vi "Parser_0x51_(SubVI).vi"(8 "error in":errorcluster, 10 "NumberTableParam":i32 format="%0d", 11 "String in":string="!01515B5461626C655D0A466F726D61743D310A4163636573733D726F0A506172616D4E756D3D300A4E616D653D54657374436170747572650A446573633D5465737420636170747572650A547970653D667261637431360A436F6C733D320A526F77733D310A4E656564506172616D507265706172653D790A466F726D61745374723D2534660A85\r") -> (0 "error out":errorcluster, 1 "CheckSummGood":bool, 3 "output cluster":T1)   [LabVIEW 2017, in "LV_Unicorn.lvlib"]
uses:
  LV_Unicorn.lvlib
  Control/unicorn_Table.ctl
panel:
  out "Array":string[][](array[string])
  out "StringOut":string
  out "CalcCheckSumm_U32":u32 format="%02x"
  out "ReciveCheckSumm_U32":i32 format="%x"
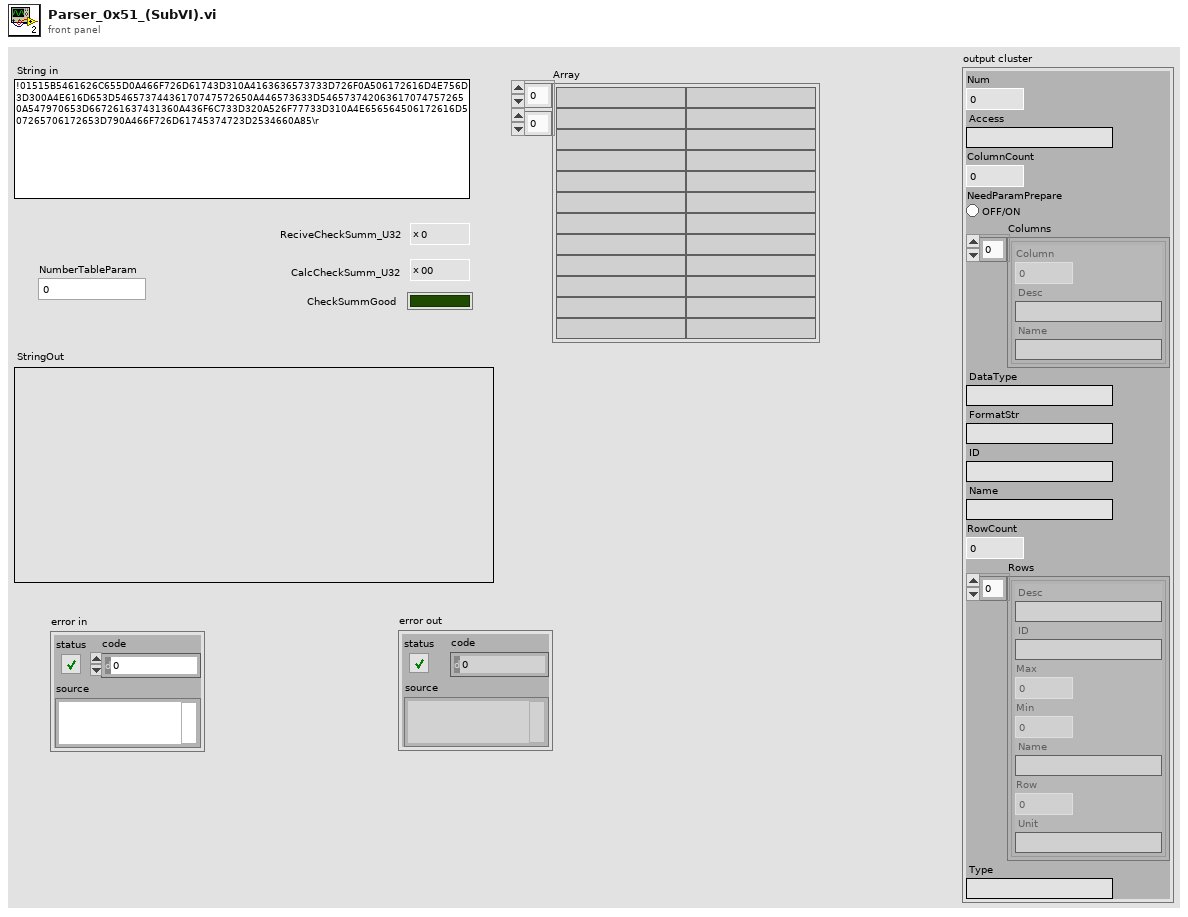
[diagram p1: front panel]
types:
  T1 = cluster{"Num":i32, "Access":string, "ColumnCount":i32, "NeedParamPrepare":bool, "Columns":cluster{"Column":i32, "Desc":string, "Name":string}[], "DataType":string, "FormatStr":string, "ID":string, "Name":string, "RowCount":i32, "Rows":cluster{"Desc":string, "ID":string, "Max":i32, "Min":i32, "Name":string, "Row":i32, "Unit":string}[], "Type":string}
  T2 = cluster{"Desc":string, "ID":string, "Max":i32, "Min":i32, "Name":string, "Row":i32, "Unit":string}[]
  T3 = cluster{"Column":i32, "Desc":string, "Name":string}[]
  T4 = typedef "LV_Unicorn.lvlib/unicorn_Table.ctl" = cluster{"Num":i32, "Access":string, "ColumnCount":i32, "NeedParamPrepare":bool, "Columns":cluster{"Column":i32, "Desc":string, "Name":string}[], "DataType":string, "FormatStr":string, "ID":string, "Name":string, "RowCount":i32, "Rows":cluster{"Desc":string, "ID":string, "Max":i32, "Min":i32, "Name":string, "Row":i32, "Unit":string}[], "Type":string}[]
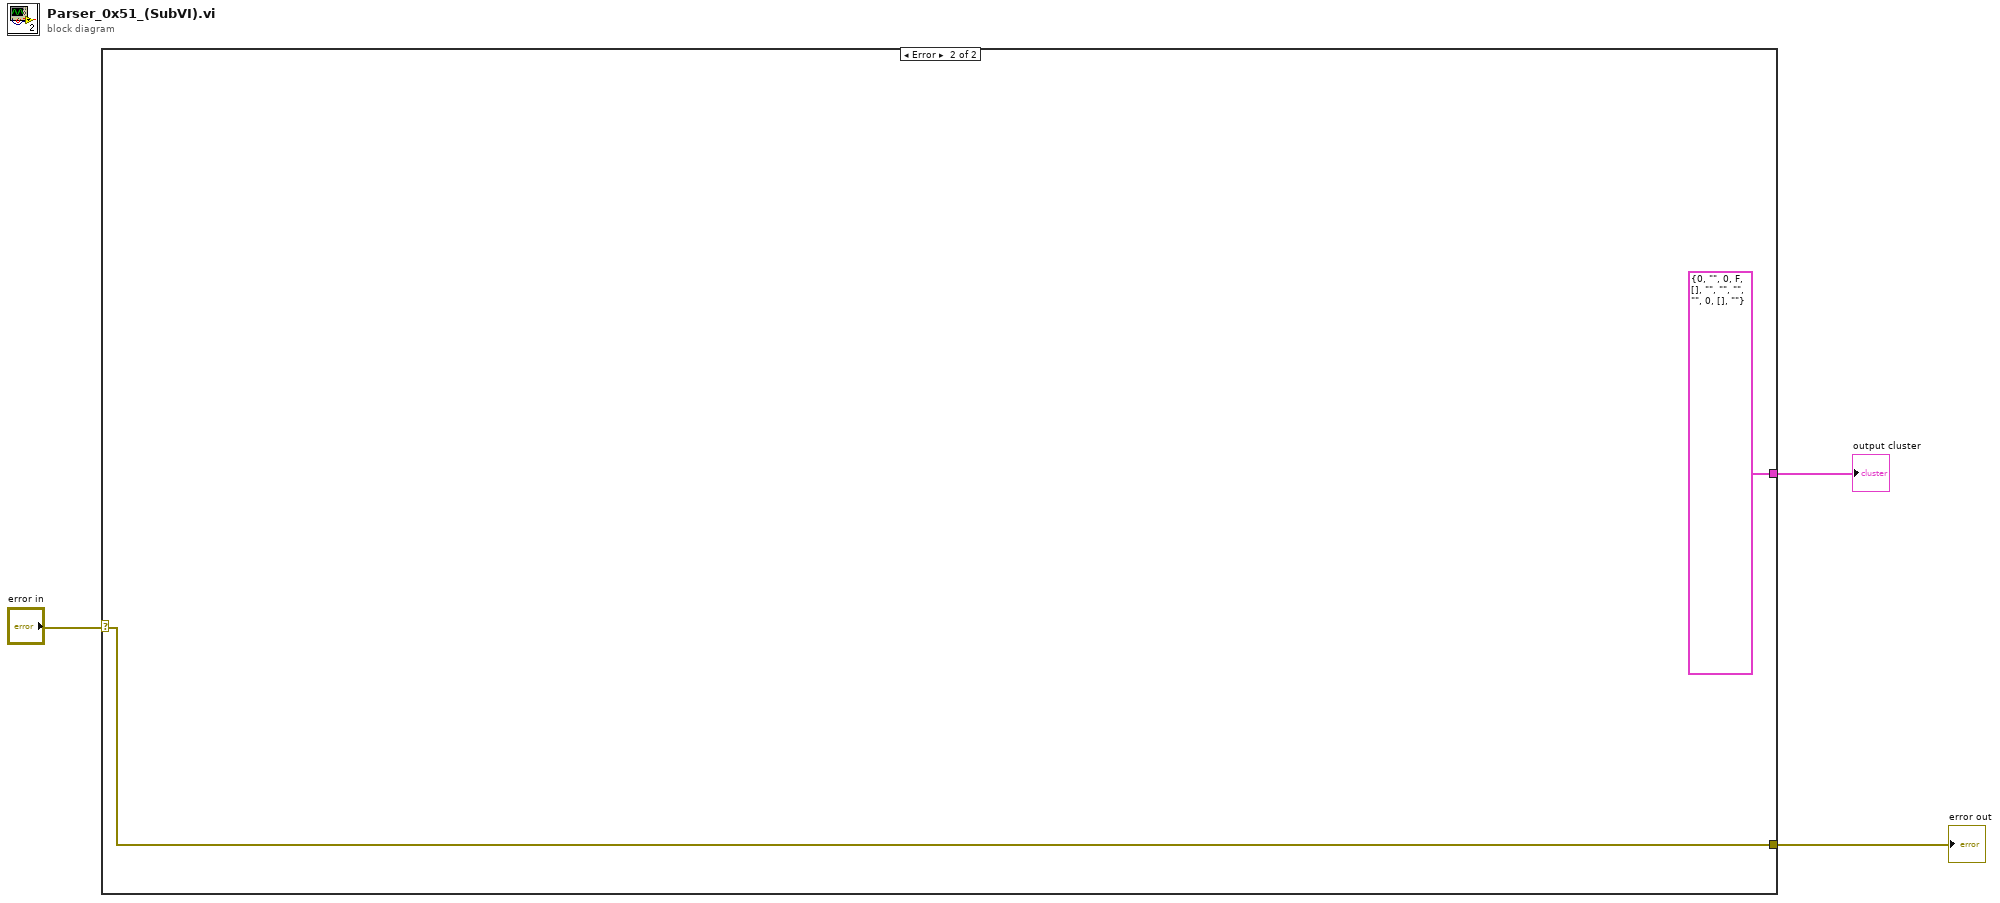
[diagram p0: block diagram]
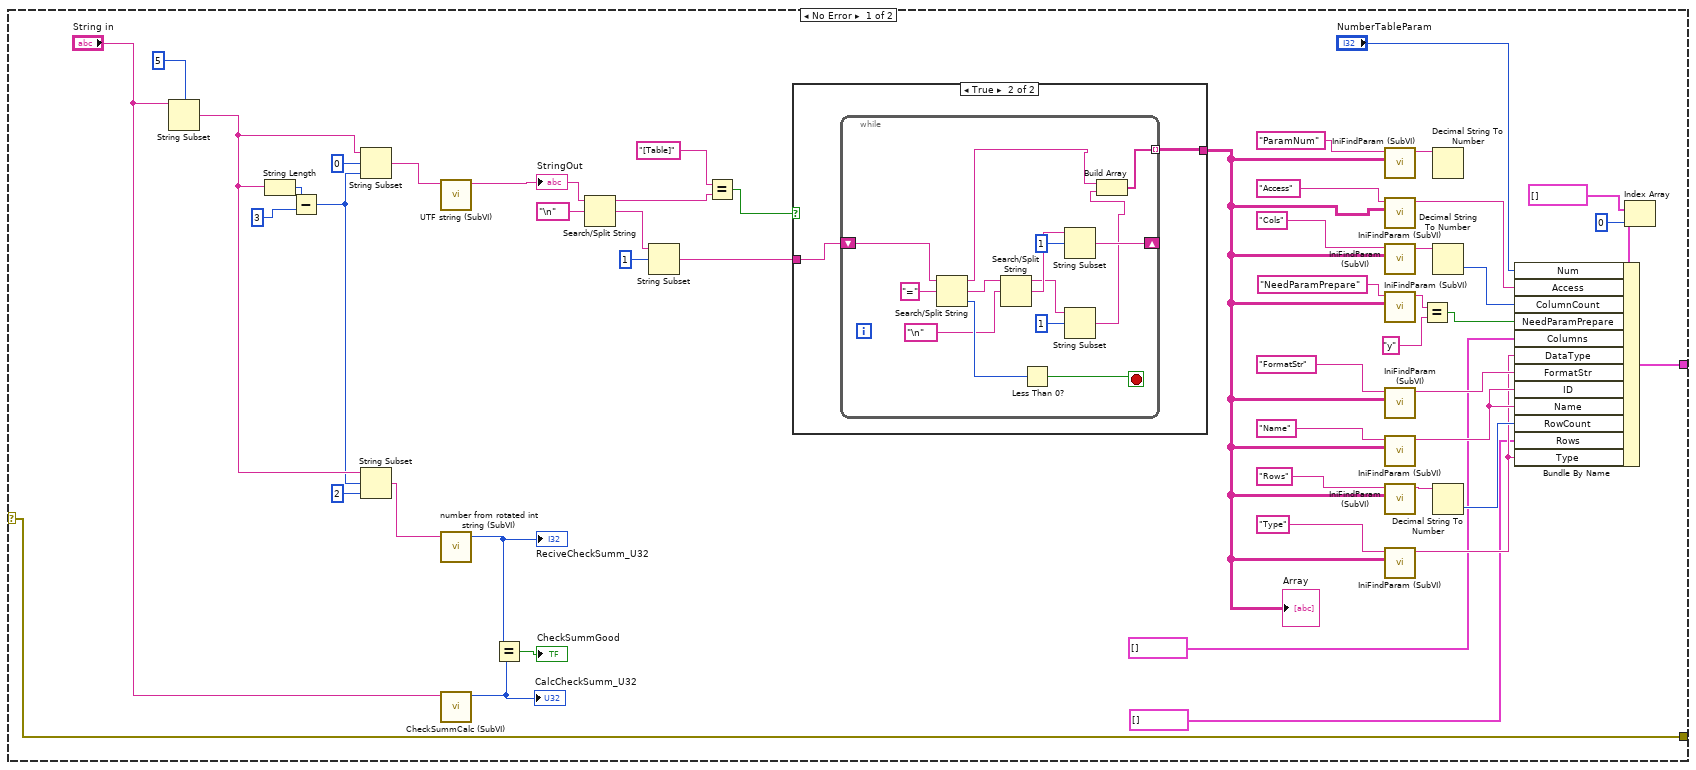
[diagram p2: hidden frame]
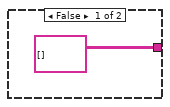
[diagram p3: hidden frame]
diagram:
  n1 = case shown="Error" "error in" {
    selector: "error in" -> [w4 w71]
    tunnel: [w18 T1 {"Num"=0, "Access"="", "ColumnCount"=0, "NeedParamPrepare"=FALSE, "Columns"=[], "DataType"="", "FormatStr"="", "ID"="", "Name"="", "RowCount"=0, "Rows"=[], "Type"=""} ("Cluster - Thin Border")] -> w3
    tunnel: [w4 w71] -> w1
    frame No Error {
      n2 = String Subset(string="String in", offset (0)=5) -> (substring=w44:string)  [unwired: 1 in]
      n3 = String Length(string=w44) -> (length=w47:i32)
      n4 = Subtract(x=w47, y=3) -> (x-y=w43:i32)
      n5 = String Subset(string=w44, offset (0)=0, length (rest)=w43) -> (substring=w45:string)
      n6 = String Subset(string=w44, offset (0)=w43, length (rest)=2 ("length (rest)")) -> (substring=w42:string)
      n7 = call "UTF string (SubVI).vi"("StringIn"=w45) -> ("StringOut"=w40:string)  [unwired: 9 in, 1 out]
      "StringOut" <- w40
      n8 = call "number from rotated int string (SubVI).vi"("String"=w42) -> ("rotated int number"=w51:i32)  [unwired: 2 in, 2 out]
      "ReciveCheckSumm_U32" <- w51
      n9 = call "CheckSummCalc (SubVI).vi"("String in"="String in") -> ("CheckSumm_U32"=w50:u32)  [unwired: 10 in]
      "CalcCheckSumm_U32" <- w50
      n10 = Equal?(x=w51, y=w50) -> (x = y?=→"CheckSummGood":bool)
      n11 = Search/Split String(string=w40, search string/char (-)="\n") -> (substring before match=w35:string, match + rest of string=w38:string)  [unwired: 1 in, 1 out]
      n12 = String Subset(string=w38, offset (0)=1) -> (substring=w33:string)  [unwired: 1 in]
      n13 = Equal?(x="[Table]" ("substring before match"), y=w35) -> (x = y?=w34:bool)
      n14 = case shown="True" w34 {
        tunnel: w33 -> [_ w56]
        tunnel: [string[][] [] w55] -> w9
        frame False {
        }
        frame True {
          n15 = while {
            shift-right: [w65] -> _
            shift-left: w56 -> [w70]
            tunnel: [w57] -> w55 mode=indexing
            stop <- w67 stop-if-true
            n16 = Search/Split String(string=w70, search string/char (-)="=") -> (substring before match=w59:string, match + rest of string=w64:string, offset of match=w68:i32)  [unwired: 1 in]
            n17 = Search/Split String(string=w64, search string/char (-)="\n") -> (substring before match=w60:string, match + rest of string=w62:string)  [unwired: 1 in, 1 out]
            n18 = Less Than 0?(x=w68) -> (x < 0?=w67:bool)
            n19 = String Subset(string=w62, offset (0)=1) -> (substring=w65:string)  [unwired: 1 in]
            n20 = String Subset(string=w60, offset (0)=1) -> (substring=w58:string)  [unwired: 1 in]
            n21 = Build Array(w59, w58) -> (w57:string[])
          }
        }
      }
      "Array" <- w9
      n22 = call "IniFindParam (SubVI).vi"("Array"=w9, "element"="ParamNum") -> ("StringOut"=w16:string)  [unwired: 9 in]
      n23 = call "IniFindParam (SubVI).vi"("Array"=w9, "element"="Access") -> ("StringOut"=w8:string)  [unwired: 9 in]
      n24 = call "IniFindParam (SubVI).vi"("Array"=w9, "element"="Cols") -> ("StringOut"=w28:string)  [unwired: 9 in]
      n25 = call "IniFindParam (SubVI).vi"("Array"=w9, "element"="NeedParamPrepare") -> ("StringOut"=w13:string)  [unwired: 9 in]
      n26 = call "IniFindParam (SubVI).vi"("Array"=w9, "element"="FormatStr") -> ("StringOut"=w20:string)  [unwired: 9 in]
      n27 = call "IniFindParam (SubVI).vi"("Array"=w9, "element"="Name") -> ("StringOut"=w22:string)  [unwired: 9 in]
      n28 = call "IniFindParam (SubVI).vi"("Array"=w9, "element"="Rows") -> ("StringOut"=w25:string)  [unwired: 9 in]
      n29 = call "IniFindParam (SubVI).vi"("Array"=w9, "element"="Type") -> ("StringOut"=w15:string)  [unwired: 9 in]
      n30 = Equal?(x=w13, y="y") -> (x = y?=w11:bool)
      n31 = Decimal String To Number(string=w16) -> ()  [unwired: 2 in, 2 out]
      n32 = Decimal String To Number(string=w28) -> (number=w27:i32)  [unwired: 2 in, 1 out]
      n33 = Decimal String To Number(string=w25) -> (number=w24:i32)  [unwired: 2 in, 1 out]
      n34 = Index Array(array=T4 [] ("Table"), index=0) -> (element=w30:T1)
      n35 = Bundle By Name(cluster=w30, "Num"="NumberTableParam", "Access"=w8, "ColumnCount"=w27, "NeedParamPrepare"=w11, "Columns"=T3 [], "DataType"=w15, "FormatStr"=w20, "ID"=w22, "Name"=w22, "RowCount"=w24, "Rows"=T2 [], "Type"=w15) -> (w18:T1)
    }
    frame Error {
    }
  }
  "output cluster" <- w3
  "error out" <- w1
